vi "Profile Step 2 Desired Parameters.vi"(0 "ProfileStep":string[](array[string]), 7 "Controller?":bool, 11 "CMD Cluster IN":T1) -> (4 "ParameterSet":string)   [LabVIEW 2013]
uses:
  TypeDef/Command Cluster.ctl
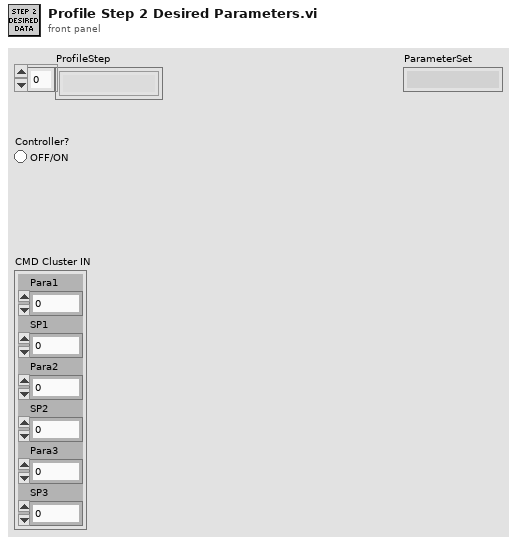
[diagram p1: front panel]
types:
  T1 = typedef "Command Cluster.ctl" = cluster{"Para1":i32, "SP1":dbl, "Para2":i32, "SP2":dbl, "Para3":i32, "SP3":dbl}
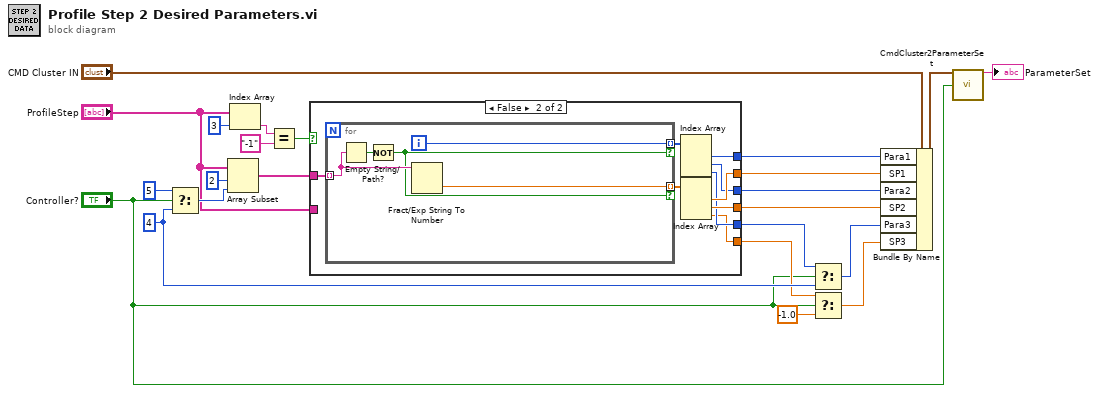
[diagram p0: block diagram]
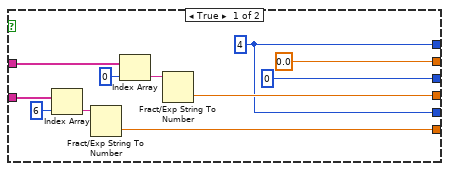
[diagram p2: hidden frame]
diagram:
  w19 = 4 ("index")
  n1 = Select(t=5 ("length"), s="Controller?", f=w19) -> (s? t:f=w15:i32)
  n2 = Array Subset(array="ProfileStep", index=2, length=w15) -> (w7:string[])
  n3 = Index Array(array="ProfileStep", index=3) -> (element=w11:string)
  n4 = Equal?(x=w11, y="-1") -> (x = y?=w13:bool)
  n5 = case shown="False" w13 {
    tunnel: w7 -> [w34 w43]
    tunnel: [0.0 w40] -> w8
    tunnel: [w31 w39] -> w9
    tunnel: [w28 w38] -> w23
    tunnel: [0 w37] -> w22
    tunnel: [w28 w36] -> w17
    tunnel: [w24 w35] -> w16
    tunnel: "ProfileStep" -> [w25 _]
    frame True {
      w28 = 4
      n6 = Index Array(array=w25, index=6) -> (element=w26:string)
      n7 = Fract/Exp String To Number(string=w26) -> (number=w24:dbl)  [unwired: 3 in, 1 out]
      n8 = Index Array(array=w34, index=0) -> (element=w32:string)
      n9 = Fract/Exp String To Number(string=w32) -> (number=w31:dbl)  [unwired: 3 in, 1 out]
    }
    frame False {
      n10 = for {
        tunnel: w43 -> [w48] mode=indexing
        tunnel: [w44] -> w42 mode=indexing if=w45
        tunnel: [w46] -> w41 mode=indexing if=w45
        i -> [w46]
        n11 = Empty String/Path?(string/path=w48) -> (empty?=w47:bool)
        n12 = Not(x=w47) -> (.not. x?=w45:bool)
        n13 = Fract/Exp String To Number(string=w48) -> (number=w44:dbl)  [unwired: 3 in, 1 out]
      }
      n14 = Index Array(array=w41) -> (element #1=w38:i32, element #2=w37:i32, element #3=w36:i32)  [unwired: 3 in]
      n15 = Index Array(array=w42) -> (element #1=w40:dbl, element #2=w39:dbl, element #3=w35:dbl)  [unwired: 3 in]
    }
  }
  n16 = Select(t=w17, s="Controller?", f=w19) -> (s? t:f=w21:i32)
  n17 = Select(t=w16, s="Controller?", f=-1.0) -> (s? t:f=w18:dbl)
  n18 = Bundle By Name(cluster="CMD Cluster IN", "Para1"=w23, "SP1"=w8, "Para2"=w22, "SP2"=w9, "Para3"=w21, "SP3"=w18) -> (w1:T1)
  n19 = call "CmdCluster2ParameterSet.vi"("CMDCluster"=w1, "Controller?"="Controller?") -> ("ParameterSet"=→"ParameterSet":string)  [unwired: 13 in]
